vi "themometer.vi"() -> ()   [LabVIEW 2017]
uses:
  <vilib>/Platform/TimedLoop/XDataNode/timing_clust.ctl
  <vilib>/Platform/TimedLoop/XDataNode/nitl_modes.ctl
  <vilib>/Platform/TimedLoop/XDataNode/wakeup.ctl
  <vilib>/DAQmx/read.llb/DAQmx Read (Analog DBL 1Chan 1Samp).vi
  <vilib>/DAQmx/write.llb/DAQmx Write (Analog DBL 1Chan 1Samp).vi
  <vilib>/DAQmx/create/channels.llb/DAQmx Create Channel (AI-Voltage-Basic).vi
  <vilib>/DAQmx/create/channels.llb/DAQmx Create Channel (AO-Voltage-Basic).vi
  <vilib>/DAQmx/miscellaneous.llb/DAQmx Fill In Error Info.vi
  <vilib>/platform/TimedLoop/XDataNode/XDataNode.xnode
  <vilib>/Platform/TimedLoop/XDataNode/XDNodeRunTimeDep.lvlib
  <vilib>/addons/control/pid/NI_PID_autopid.lvlib
panel:
  in  "autotune? (F)":bool
  out "Autotuning PID gains out":T1={"proportional gain (Kc)"=1.0, "integral time (Ti, min)"=0.01, "derivative time (Td, min)"=0.0} {"derivative time (Td, min)" format="%.3f"; "integral time (Ti, min)" format="%.3f"; "proportional gain (Kc)" format="%.3f"}
  in  "autotuning parameters":T2={"controller type"=1, "relay cycles"=3, "relay amplitude"=1.0, "control specification"=2, "PV noise level"=0.1} {"PV noise level" format="%.2f"; "control specification" items=["normal", "fast", "slow"]; "relay amplitude" format="%.2f"; "controller type" items=["PID", "PI", "P"]}
  in  "Temperature \nupdate period ms":i64=10
  out "Heater voltage":dbl format="%.2f"
  in  "PID gains":T1={"proportional gain (Kc)"=0.398, "integral time (Ti, min)"=0.01577, "derivative time (Td, min)"=0.0} {"derivative time (Td, min)" format="%.3f"; "integral time (Ti, min)" format="%.3f"; "proportional gain (Kc)" format="%.3f"}
  in  "setpoint":dbl format="%.2f"
  out "temp":dbl(graph)
  out "Temp C":dbl
  in  "stop":bool
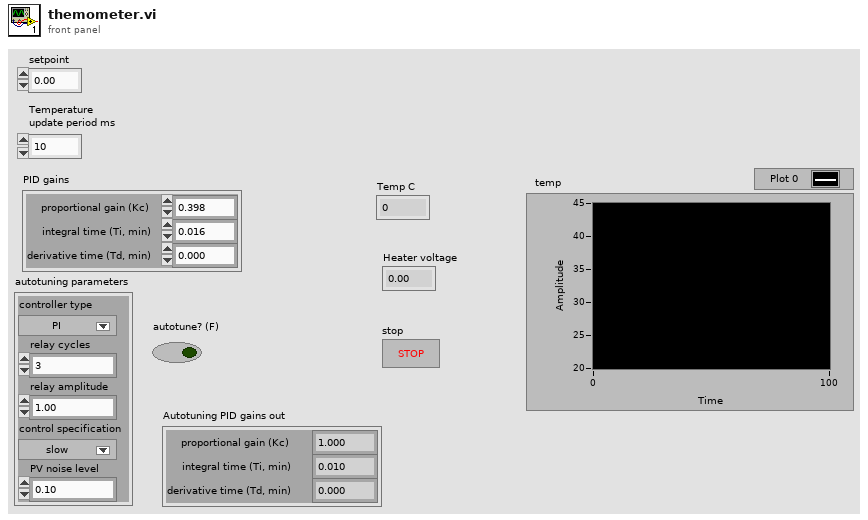
[diagram p1: front panel]
types:
  T1 = cluster{"proportional gain (Kc)":dbl, "integral time (Ti, min)":dbl, "derivative time (Td, min)":dbl}
  T2 = cluster{"controller type":u16, "relay cycles":i32, "relay amplitude":dbl, "control specification":u16, "PV noise level":dbl}
  T3 = typedef "XDNodeRunTimeDep.lvlib/timing_clust.ctl" = cluster{"Expected End [f-1]":u64, "Actual End [f-1]":u64, "Finished Late? [f-1]":bool, "Expected End [i-1]":u64, "Actual End [i-1]":u64, "Finished Late? [i-1]":bool, "Expected Start [i]":u64, "Actual Start [i]":u64, "Expected Start [f]":u64, "Actual Start [f]":u64, "Source Name":string, "Structure Name":string, "Period":i64, "Deadline":i64, "Offset":i64, "Start":i64, "Priority":i32, "Timeout":i32, "Mode":T4, "Wakeup Reason":T5, "Error":errorcluster, "Source Type":string, "Secondary Source Type":string, "Global End Time":u64, "Global Start Time":u64, "Frame Duration":u64, "Iteration Duration":u64, "Assigned CPU":i32, "I/O Scan Engine Mode":u32}
  T4 = typedef "XDNodeRunTimeDep.lvlib/nitl_modes.ctl" = enum32{"No Change", "Process missed periods, maintain original phase", "Discard missed periods, maintain original phase", "Process missed periods, ignore original phase", "Discard missed periods, ignore original phase"}
  T5 = typedef "XDNodeRunTimeDep.lvlib/wakeup.ctl" = enum32{"Normal", "Aborted", "Asynchronous wakeup", "Timing source error", "Timed loop error", "Timeout"}
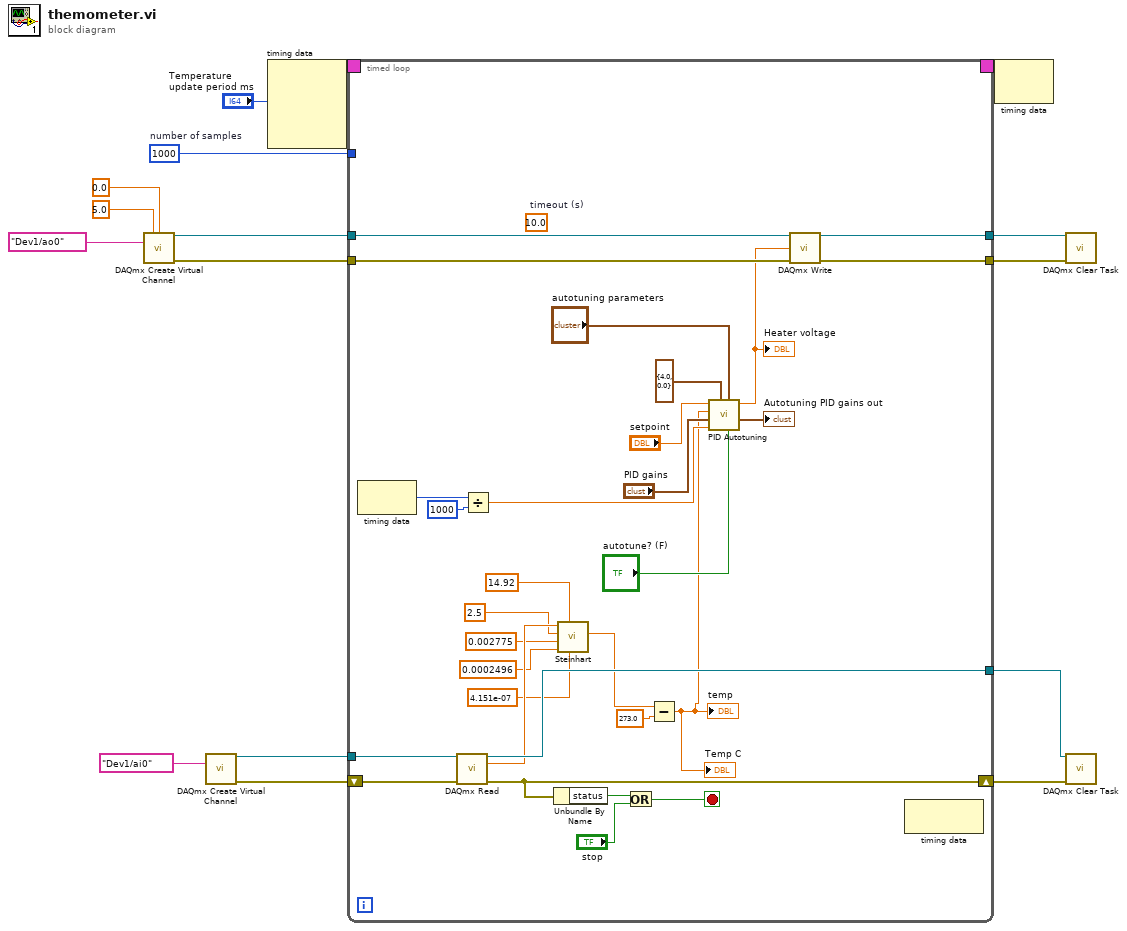
[diagram p0: block diagram]
diagram:
  w16 = 1000  # number of samples
  n1 = call-poly <vilib>:"DAQmx Create Virtual Channel.vi"("maximum value"=5.0, "minimum value"=0.0, "physical channels"=tag "Dev1/ao0") -> ("task out"=w11:refnum<k21>, "error out"=w9:errorcluster)  [unwired: 11 in]
  n2 = call-poly <vilib>:"DAQmx Create Virtual Channel.vi"("physical channels"=tag "Dev1/ai0") -> ("task out"=w5:refnum<k21>, "error out"=w4:errorcluster)  [unwired: 13 in]
  n3 = node-c288("Temperature \nupdate period ms") -> (w3:T3)  [unwired: 3 in]
  n4 = timed-loop {
    tunnel: w5 -> [w43]
    tunnel: w16 -> [_]
    tunnel: [w42] -> w14
    shift-right: [w40] -> w15
    shift-left: w4 -> [w41]
    tunnel: w11 -> [w31]
    tunnel: [w30] -> w10
    tunnel: w9 -> [w29]
    tunnel: [w28] -> w8
    timing: w3 -> [_]
    timing-out: [_] -> w2
    stop <- w45 stop-if-true
    (unwired) 10.0  # timeout (s)
    n5 = node-c288() -> (w27:i64)  [unwired: 1 in]
    n6 = call-poly <vilib>:"DAQmx Read.vi"("task/channels in"=w43, "error in"=w41) -> ("task out"=w42:refnum<k21>, "data"=w39:dbl, "error out"=w40:errorcluster)  [unwired: 11 in]
    n7 = Divide(x=w27, y=i64 1000) -> (x/y=w24:dbl)
    n8 = Unbundle By Name(w40) -> ("status"=w46:bool)
    n9 = call "Steinhart.vi"("c"=4.151e-07, "R1"=14.92, "b"=0.0002496, "a"=0.002775, "Vex"=2.5, "Vm"=w39) -> ("output variable"=w34:dbl)  [unwired: 5 in]
    n10 = Or(x=w46, y="stop") -> (x .or. y?=w45:bool)
    n11 = Subtract(x=w34, y=273.0) -> (x-y=w17:dbl)
    "Temp C" <- w17
    "temp" <- w17
    n12 = call <vilib>:"PID Autotuning.vi"("autotune? (F)"="autotune? (F)", "autotuning parameters"="autotuning parameters", "output range"=cluster{"output high":dbl, "output low":dbl} {"output high"=4.0, "output low"=0.0}, "dt (s)"=w24, "PID gains"="PID gains", "process variable"=w17, "setpoint"="setpoint") -> ("PID gains out"=→"Autotuning PID gains out":T1, "output"=w20:dbl)  [unwired: 1 in, 2 out]
    "Heater voltage" <- w20
    n13 = call-poly <vilib>:"DAQmx Write.vi"("task/channels in"=w31, "data"=w20, "error in"=w29) -> ("task out"=w30:refnum<k21>, "error out"=w28:errorcluster)  [unwired: 10 in, 1 out]
    n14 = node-c288() -> ()  [unwired: 1 in, 1 out]
  }
  n15 = node-c288(w2) -> ()  [unwired: 1 out]
  n16 = call <vilib>:"DAQmx Clear Task.vi"("task in"=w10, "error in"=w8) -> ()  [unwired: 13 in, 1 out]
  n17 = call <vilib>:"DAQmx Clear Task.vi"("task in"=w14, "error in"=w15) -> ()  [unwired: 13 in, 1 out]
